vi "Porównanie stanu powietrza1.vi"() -> ()   [LabVIEW 2024]
panel:
  out "Stan powietrza":string
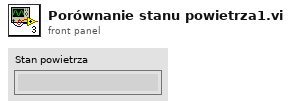
[diagram p1: front panel]
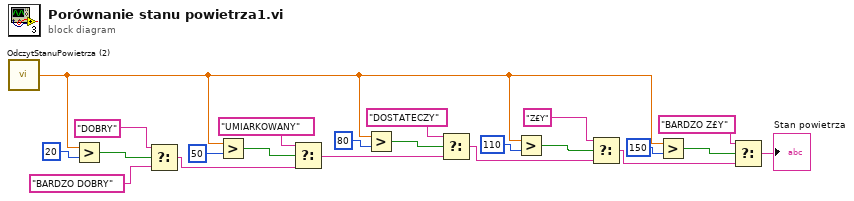
[diagram p0: block diagram]
diagram:
  n1 = call "OdczytStanuPowietrza (2).vi"() -> ("Wartoœæ"=w6:dbl)
  n2 = Greater?(x=w6, y=20) -> (0:w5:bool)
  n3 = Select(t="DOBRY", s=w5, f="BARDZO DOBRY") -> (s? t:f=w8:string)
  n4 = Greater?(x=w6, y=50) -> (0:w4:bool)
  n5 = Select(t="UMIARKOWANY", s=w4, f=w8) -> (s? t:f=w18:string)
  n6 = Greater?(x=w6, y=80) -> (0:w3:bool)
  n7 = Select(t="DOSTATECZY", s=w3, f=w18) -> (s? t:f=w15:string)
  n8 = Greater?(x=w6, y=110) -> (0:w1:bool)
  n9 = Select(t="Z£Y", s=w1, f=w15) -> (s? t:f=w11:string)
  n10 = Greater?(x=w6, y=150) -> (0:w2:bool)
  n11 = Select(t="BARDZO Z£Y", s=w2, f=w11) -> (s? t:f=→"Stan powietrza":string)
